vi "Generador de funciones.vi"() -> ()   [LabVIEW 2025]
uses:
  <vilib>/measure/NI_MABase.lvlib
panel:
  in  "Pin":u8=25 min=25 max=26
  out "error out":errorcluster
  in  "VISA resource name":refnum<visa-resource-name>
  out "Waveform Chart 3":u8(graph)
  in  "Unidad":u16(ring) items=["Valor DAC", "Voltaje"]
  in  "duty cycle (%)":dbl=50.0 format="%0.2f"
  in  "Seleccion":u16(ring) items=["Cuadrada", "Senoidal", "Diente de sierra", "Triangular"]
  in  "stop":bool
  out "Valor DAC / Voltaje":dbl
  in  "F":u32
  # "Generador de Funciones   LV_ESP32"
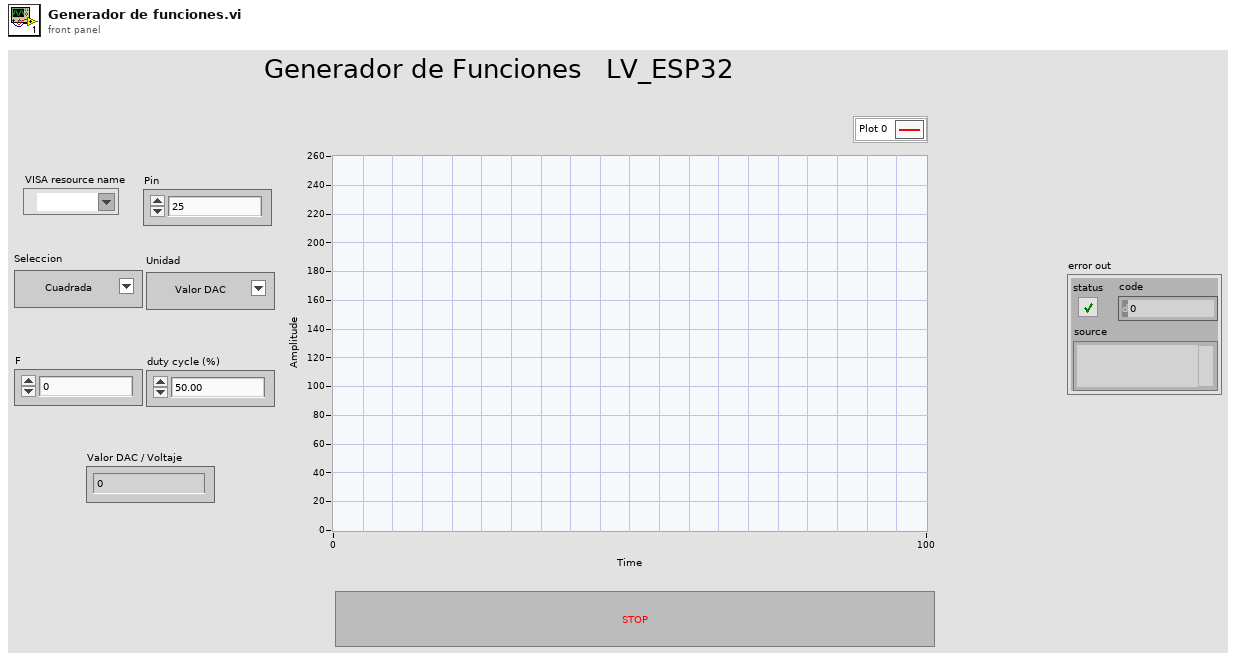
[diagram p1: front panel]
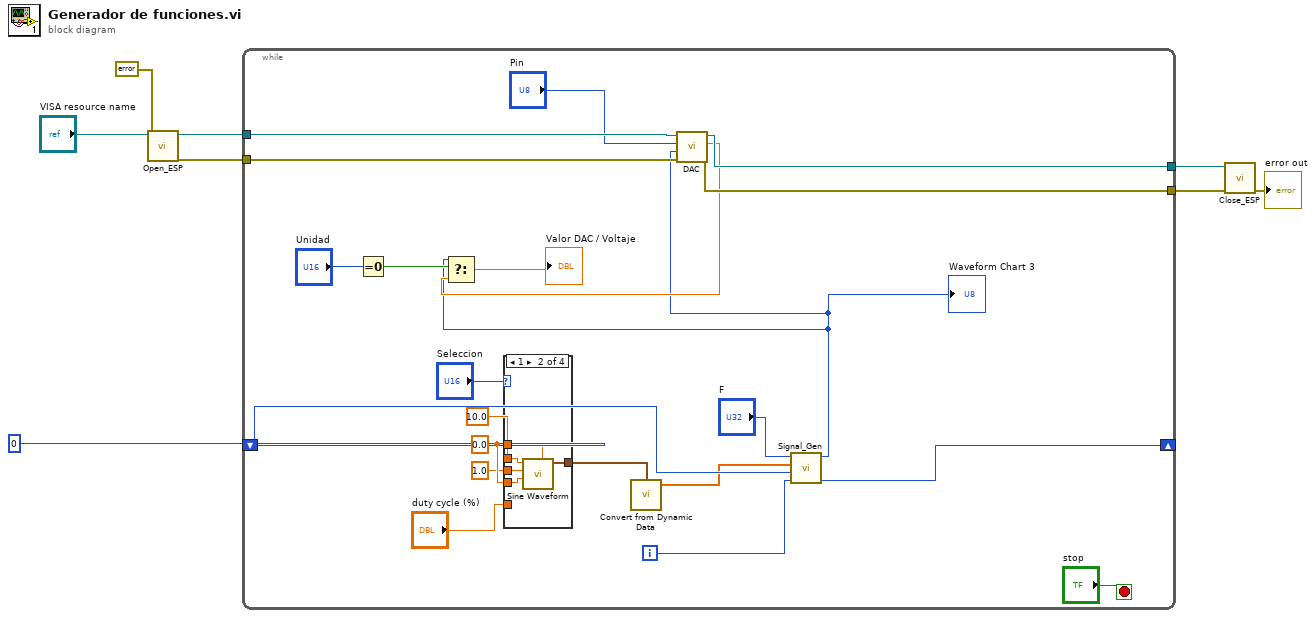
[diagram p0: block diagram]
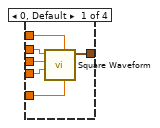
[diagram p2: hidden frame]
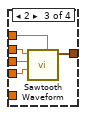
[diagram p3: hidden frame]
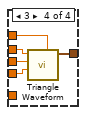
[diagram p4: hidden frame]
diagram:
  n1 = call "Open_ESP.vi"("error in (no error)"=errorcluster {"status"=FALSE, "code"=0, "source"=""}, "VISA resource name"="VISA resource name") -> ("error out"=w4:errorcluster, "VISA resource name out"=w7:refnum<visa-resource-name>)  [unwired: 8 in]
  n2 = while {
    shift-right: [w28] -> _
    shift-left: u32 0 ("timeout (10sec)") -> [w27]
    tunnel: w7 -> [w18]
    tunnel: [w17] -> w6
    tunnel: [w16] -> w5
    tunnel: w4 -> [w15]
    i -> [w29]
    stop <- "stop" stop-if-true
    w22 = 0.0
    n3 = Equal To 0?(x="Unidad") -> (x = 0?=w13:bool)
    n4 = case shown="1" "Seleccion" {
      tunnel: [w36 w41 w46 w51] -> w19
      tunnel: w22 -> [w32 w40 w42 w47]
      tunnel: w22 -> [w33 w39 w43 w48]
      tunnel: 1.0 -> [w34 w38 w44 w49]
      tunnel: 10.0 -> [w35 w37 w45 w50]
      tunnel: "duty cycle (%)" -> [w31 _ _ _]
      frame 0, Default {
        n5 = call <vilib>:"Square Waveform.vi"("duty cycle (%)"=w31, "offset"=w32, "phase"=w33, "amplitude"=w34, "frequency"=w35) -> ("signal out"=w36:waveform(dbl))  [unwired: 5 in, 1 out]
      }
      frame 1 {
        n6 = call <vilib>:"Sine Waveform.vi"("offset"=w40, "phase"=w39, "amplitude"=w38, "frequency"=w37) -> ("signal out"=w41:waveform(dbl))  [unwired: 6 in, 1 out]
      }
      frame 2 {
        n7 = call <vilib>:"Sawtooth Waveform.vi"("offset"=w42, "phase"=w43, "amplitude"=w44, "frequency"=w45) -> ("signal out"=w46:waveform(dbl))  [unwired: 6 in, 1 out]
      }
      frame 3 {
        n8 = call <vilib>:"Triangle Waveform.vi"("offset"=w47, "phase"=w48, "amplitude"=w49, "frequency"=w50) -> ("signal out"=w51:waveform(dbl))  [unwired: 6 in, 1 out]
      }
    }
    n9 = call "Convert from Dynamic Data"("Dynamic Data Type"=w19) -> ("Array"=w25:dbl[])  [unwired: 3 in]
    n10 = call "Signal_Gen.vi"("Iteraciones"=w29, "entrada"=w27, "Entrada"=w25, "F"="F") -> ("salida_shift_reg"=w28:i64, "Salida"=w9:u8)  [unwired: 6 in]
    "Waveform Chart 3" <- w9
    n11 = call "DAC.vi"("error in (no error)"=w15, "DAC"=w9, "Pin"="Pin", "VISA resource name"=w18) -> ("error out"=w16:errorcluster, "Voltaje"=w12:dbl, "VISA resource name out"=w17:refnum<visa-resource-name>)  [unwired: 5 in]
    n12 = Select(t=w9, s=w13, f=w12) -> (s? t:f=→"Valor DAC / Voltaje":dbl)
  }
  n13 = call "Close_ESP.vi"("error in (no error)"=w5, "VISA resource name"=w6) -> ("error out"=→"error out":errorcluster)  [unwired: 9 in]
